vi "Update Worktable Fid Positions.vi"(8 "error in":errorcluster, 11 "Gluing Procedure in":refnum<class "Gluing Procedure.lvclass">) -> (0 "error out":errorcluster, 3 "Gluing Procedure out":refnum<class "Gluing Procedure.lvclass">)   [LabVIEW 2017, in "Gluing Procedure.lvclass"]
uses:
  Procedure Classes/Gluing Procedure/Gluing Procedure.lvclass
  Shared Components/Gantry Class/Gantry Class.lvclass
  Shared Components/Config Manager Class/Config Manager Class.lvclass
  Shared Components/Config Manager Class/Type Definitions/Fiducial Type.ctl
  Shared Components/WorkTable Class/WorkTable Class.lvclass
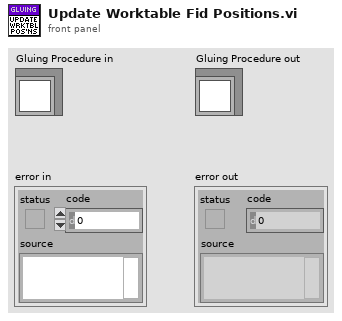
[diagram p1: front panel]
types:
  T1 = typedef "Fiducial Type.ctl" = enum16{"HDI", "BBM"}
  T2 = typedef "Inspect Fuducials.ctl" = cluster{"Path Fiducials":cluster{"HDI Fiducials":T3, "Stamp Fiducials":T3, "Weight Fiducials":T3, "BBM Fiducials":T3}[], "Has been run?":bool}
  T3 = typedef "Part Fiducials.ctl" = cluster{"Fiducials":T4[], "Chuck":i32, "Slot":i32}
  T4 = typedef "Fiducial Image.ctl" = cluster{"Fiducial Image":T5, "Selected Fiducial":T7, "fiducial name":string}
  T5 = typedef "Physical Image.ctl" = cluster{"Image Position":refnum<class "Vec3d Class.lvclass">, "Image Reference":T6, "Field of View":cluster{"x(mm)":dbl, "y(mm)":dbl}}
  T6 = typedef "IMAQ Image.ctl" = refnum<image>
  T7 = typedef "Fiducial with Source.ctl" = cluster{"Fiducial Image Coordinate":refnum<class "Vec3d Class.lvclass">, "Fiducial Source":enum16{"Pattern Recognition", "User", "Error", "Default"}}
  T8 = cluster{"HDI Fiducials":T3, "Stamp Fiducials":T3, "Weight Fiducials":T3, "BBM Fiducials":T3}[]
  T9 = cluster{"Feature Coordinates":refnum<class "Vec3d Class.lvclass">, "Feature Name":string}[]
  T10 = typedef "Position_Orientation.ctl" = cluster{"Center":refnum<class "Vec3d Class.lvclass">, "Orientation":refnum<class "Orient3d Class.lvclass">}
  T11 = typedef "Worktable_Module Slot.ctl" = cluster{"Slot State":enum16{"Empty", "Bare HDI", "Unglued", "Stamped", "PartOnTop", "Weighted", "Unpotted", "Potted"}, "BBM Type":enum16{"None", "BBM", "GlassSlide"}, "HDI Type":enum16{"None", "HDI", "Polyimide"}, "Vacuum Channel":u8, "Location/Orientation BBM":T10, "Location/Orientation HDI":T10, "S/N":string}
  T12 = typedef "Worktable_Stamp.ctl" = cluster{"Stamp State":enum16{"Empty", "Populated", "Used"}, "Location/Orientation":T10, "Stamp Type":T13}
  T13 = typedef "Stamp Type.ctl" = enum16{"Stamp 1", "Stamp 2", "Stamp 3", "Stamp 4", "Stamp 5"}
  T14 = typedef "Worktable_Weight.ctl" = cluster{"Weight State":enum16{"Empty", "Populated"}, "Weight Type":T15, "Location/Orientation":T10}
  T15 = typedef "Weight Type.ctl" = enum16{"Weight 1", "Weight 2", "Weight 3", "Weight 4", "Weight 5", "Weight 6", "Weight 7", "Weight 8"}
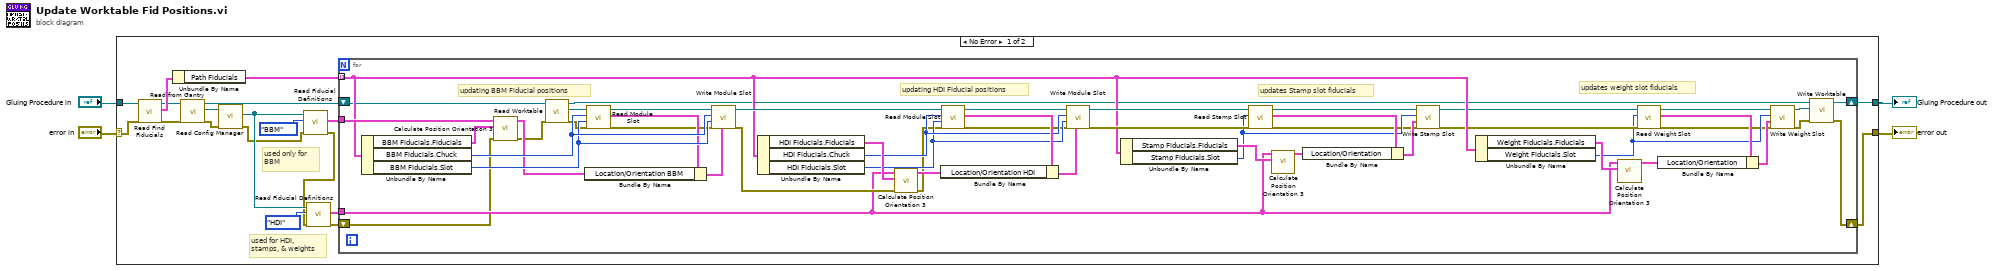
[diagram p0: block diagram]
diagram:
  n1 = case shown="No Error" "error in" {
    selector: "error in" -> [w13 w75]
    tunnel: [w7 w75] -> w3
    tunnel: [w8 w74] -> w1
    tunnel: "Gluing Procedure in" -> [w23 w74]
    frame No Error {
      # "used for HDI,\nstamps, & weights"
      # "used only for \nBBM"
      n2 = call "Read Find Fiducials.vi"("error in (no error)"=w13, "Gluing Procedure in"=w23) -> ("error out"=w12:errorcluster, "Find Fiducials"=w22:T2, "Gluing Procedure out"=w21:refnum<class "Gluing Procedure.lvclass">)  [unwired: 7 in]
      n3 = Unbundle By Name(w22) -> ("Path Fiducials"=w16:T8)
      n4 = call "Read from Gantry.vi"("error in (no error)"=w12, "Gluing Procedure in"=w21) -> ("error out"=w11:errorcluster, "Gantry"=w20:refnum<class "Gantry Class.lvclass">, "Gluing Procedure out"=w6:refnum<class "Gluing Procedure.lvclass">)  [unwired: 7 in]
      n5 = call-dynamic "Read Config Manager.vi"("error in"=w11, "Gantry in"=w20) -> ("error out"=w10:errorcluster, "Config Manager"=w17:refnum<class "Config Manager Class.lvclass">)  [unwired: 7 in, 1 out]
      n6 = call "Read Fiducial Definitions.vi"("error in"=w10, "Fiducial Type"=Fiducial_Type."BBM", "Config Manager in"=w17) -> ("error out"=w9:errorcluster, "Feature Definitions"=w15:T9)  [unwired: 6 in, 1 out]
      n7 = call "Read Fiducial Definitions.vi"("error in"=w9, "Fiducial Type"=Fiducial_Type."HDI", "Config Manager in"=w17) -> ("error out"=w5:errorcluster, "Feature Definitions"=w14:T9)  [unwired: 6 in, 1 out]
      n8 = for {
        tunnel: w16 -> [w41] mode=indexing
        tunnel: w15 -> [w73]
        tunnel: w14 -> [w39]
        shift-right: [w28] -> w8
        shift-left: w6 -> [w25]
        shift-right: [w27] -> w7
        shift-left: w5 -> [w24]
        # "updates weight slot fiducials"
        # "updates Stamp slot fiducials"
        # "updating HDI Fiducial positions"
        # "updating BBM Fiducial positions"
        n9 = Unbundle By Name(w41) -> ("BBM Fiducials.Fiducials"=w72:T4[], "BBM Fiducials.Chuck"=w69:i32, "BBM Fiducials.Slot"=w68:i32)
        n10 = call "Calculate Position Orientation 3.vi"("error in"=w24, "Fiducials"=w72, "Feature Definitions"=w73) -> ("error out"=w56:errorcluster, "PositionOrientation"=w66:T10)  [unwired: 7 in]
        n11 = call "Read Worktable.vi"("error in"=w56, "Gluing Procedure in"=w25) -> ("error out"=w55:errorcluster, "WorkTable out"=w71:refnum<class "WorkTable Class.lvclass">, "Gluing Procedure out"=w29:refnum<class "Gluing Procedure.lvclass">)  [unwired: 7 in]
        n12 = call-dynamic "Read Module Slot.vi"("error in"=w55, "slot"=w68, "chuck"=w69, "WorkTable in"=w71) -> ("error out"=w54:errorcluster, "Module Slot"=w67:T11, "WorkTable out"=w70:refnum<class "WorkTable Class.lvclass">)  [unwired: 5 in]
        n13 = Bundle By Name(cluster=w67, "Location/Orientation BBM"=w66) -> (w65:T11)
        n14 = call-dynamic "Write Module Slot.vi"("Module Slot"=w65, "error in"=w54, "slot"=w68, "chuck"=w69, "WorkTable in"=w70) -> ("error out"=w53:errorcluster, "WorkTable out"=w59:refnum<class "WorkTable Class.lvclass">)  [unwired: 5 in]
        n15 = Unbundle By Name(w41) -> ("HDI Fiducials.Fiducials"=w64:T4[], "HDI Fiducials.Chuck"=w58:i32, "HDI Fiducials.Slot"=w57:i32)
        n16 = call "Calculate Position Orientation 3.vi"("error in"=w53, "Fiducials"=w64, "Feature Definitions"=w39) -> ("error out"=w52:errorcluster, "PositionOrientation"=w60:T10)  [unwired: 7 in]
        n17 = call-dynamic "Read Module Slot.vi"("error in"=w52, "slot"=w57, "chuck"=w58, "WorkTable in"=w59) -> ("error out"=w51:errorcluster, "Module Slot"=w62:T11, "WorkTable out"=w61:refnum<class "WorkTable Class.lvclass">)  [unwired: 5 in]
        n18 = Bundle By Name(cluster=w62, "Location/Orientation HDI"=w60) -> (w63:T11)
        n19 = call-dynamic "Write Module Slot.vi"("Module Slot"=w63, "error in"=w51, "slot"=w57, "chuck"=w58, "WorkTable in"=w61) -> ("error out"=w48:errorcluster, "WorkTable out"=w49:refnum<class "WorkTable Class.lvclass">)  [unwired: 5 in]
        n20 = Unbundle By Name(w41) -> ("Stamp Fiducials.Fiducials"=w50:T4[], "Stamp Fiducials.Slot"=w45:i32)
        n21 = call "Read Stamp Slot.vi"("error in (no error)"=w48, "Stamp Slot"=w45, "WorkTable Class in"=w49) -> ("error out"=w43:errorcluster, "Stamp Slot"=w47:T12, "WorkTable Class out"=w44:refnum<class "WorkTable Class.lvclass">)  [unwired: 6 in]
        n22 = call "Calculate Position Orientation 3.vi"("Fiducials"=w50, "Feature Definitions"=w39) -> ("PositionOrientation"=w42:T10)  [unwired: 8 in, 1 out]
        n23 = Bundle By Name(cluster=w47, "Location/Orientation"=w42) -> (w46:T12)
        n24 = call "Write Stamp Slot.vi"("error in (no error)"=w43, 9:"Stamp Slot"=w46, 10:"Stamp Slot"=w45, "WorkTable Class in"=w44) -> ("error out"=w37:errorcluster, "WorkTable Class out"=w38:refnum<class "WorkTable Class.lvclass">)  [unwired: 6 in]
        n25 = Unbundle By Name(w41) -> ("Weight Fiducials.Fiducials"=w40:T4[], "Weight Fiducials.Slot"=w32:i32)
        n26 = call "Calculate Position Orientation 3.vi"("Fiducials"=w40, "Feature Definitions"=w39) -> ("PositionOrientation"=w35:T10)  [unwired: 8 in, 1 out]
        n27 = call "Read Weight Slot.vi"("error in (no error)"=w37, "weight slot"=w32, "WorkTable Class in"=w38) -> ("error out"=w31:errorcluster, "Weight Slot"=w36:T14, "WorkTable Class out"=w33:refnum<class "WorkTable Class.lvclass">)  [unwired: 6 in]
        n28 = Bundle By Name(cluster=w36, "Location/Orientation"=w35) -> (w34:T14)
        n29 = call "Write Weight Slot.vi"("error in (no error)"=w31, "Weight Slot"=w34, "weight slot"=w32, "WorkTable Class in"=w33) -> ("error out"=w26:errorcluster, "WorkTable Class out"=w30:refnum<class "WorkTable Class.lvclass">)  [unwired: 6 in]
        n30 = call "Write Worktable.vi"("error in"=w26, "WorkTable"=w30, "Gluing Procedure in"=w29) -> ("error out"=w27:errorcluster, "Gluing Procedure out"=w28:refnum<class "Gluing Procedure.lvclass">)  [unwired: 7 in]
      }
    }
    frame Error {
    }
  }
  "error out" <- w3
  "Gluing Procedure out" <- w1
